vi "Device Close.vi"(0 "VISA Rresource Name":refnum<visa-resource-name>, 11 "Error In":errorcluster) -> (15 "Error Out":errorcluster)   [LabVIEW 2025]
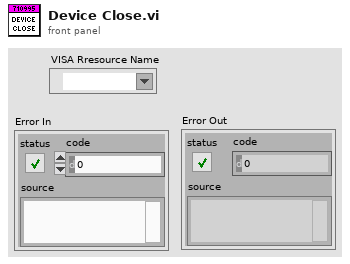
[diagram p1: front panel]
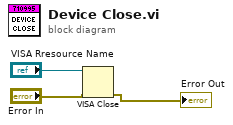
[diagram p0: block diagram]
diagram:
  n1 = VISA Close(VISA resource name="VISA Rresource Name", error in (no error)="Error In") -> (error out=→"Error Out":errorcluster)
